vi "Release-buffers.vi"(8 "error in":errorcluster, 11 "Data ref. in":refnum<data-value>) -> (0 "error IO":errorcluster, 3 "Data ref.":refnum<data-value>, 5 "Succes?":bool)   [LabVIEW 2013, in "CameraVision.lvlib" / "CV-Main.lvclass"]
doc: "This function flushes the strictly acquisition related buffers. These are currently the 'Camera' and 'CameraTime' queues and the image queue buffer.\n\nThe 'Success' output indicates no errors were produced during the flushing."
uses:
  CV-Main.lvclass
  CV-Main.lvclass/CV-Main.ctl
  Read Buffers.vi
  Buffers/CV-Buffers.lvclass
  Errors/CV-Errors.lvclass
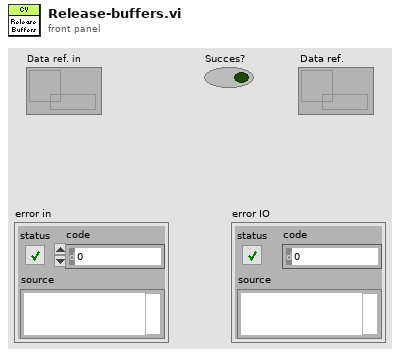
[diagram p1: front panel]
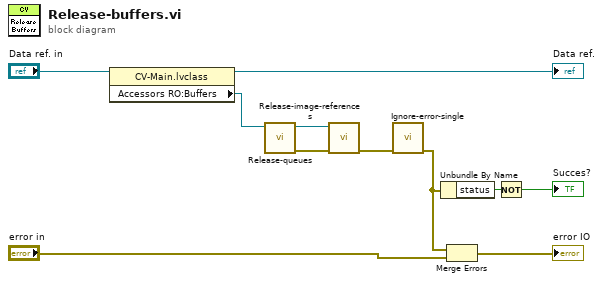
[diagram p0: block diagram]
diagram:
  n1 = property class="CV-Main.lvclass"(reference="Data ref. in") -> (reference out=→"Data ref.":refnum<data-value>, "Accessors RO:Buffers"=w2:refnum<class "CV-Buffers.lvclass">)  [unwired: 1 in, 1 out]
  n2 = call "Release-queues.vi"("Buffers in"=w2) -> ("error out"=w3:errorcluster, "Buffers out"=w1:refnum<class "CV-Buffers.lvclass">)  [unwired: 9 in]
  n3 = call "Release-image-references.vi"("error in (no error)"=w3, "Buffers in"=w1) -> ("error out"=w4:errorcluster)  [unwired: 8 in, 1 out]
  n4 = call "Ignore-error-single.vi"("error in (no error)"=w4) -> ("error out"=w5:errorcluster)  [unwired: 10 in]
  n5 = Unbundle By Name(w5) -> ("status"=w8:bool)
  n6 = Merge Errors(w5, "error in") -> (→"error IO":errorcluster)
  n7 = Not(x=w8) -> (.not. x?=→"Succes?":bool)
